vi "Config Trig Template.vi"(4 "Card Position":enum16{"Master", "Slave"}(ring), 6 "Trigger Type":enum16{"Immediate", "Analog Edge"}(ring), 8 "error in (no error)":errorcluster, 11 "4300 in":refnum<class "4300.lvclass">) -> (0 "error out":errorcluster, 3 "4300 out":refnum<class "4300.lvclass">)   [LabVIEW 2016]
uses:
  <resource>/objmgr/daqmx.rc
  Desktop/Built/AnalogInput.lvlibp/AnalogInput.lvclass
  <vilib>/DAQmx/configure/trigger.llb/DAQmx Reference Trigger (Digital Edge).vi
  <vilib>/DAQmx/configure/events/hardwareSignals.llb/DAQmx Export Signal (Most Signals).vi
  <vilib>/DAQmx/configure/trigger.llb/DAQmx Reference Trigger (None).vi
  <vilib>/DAQmx/configure/trigger.llb/DAQmx Reference Trigger (Analog Edge).vi
  4300.lvclass
  C:/Users/rdexter/Desktop/Built/AnalogInput.lvlibp/AnalogInput.lvclass
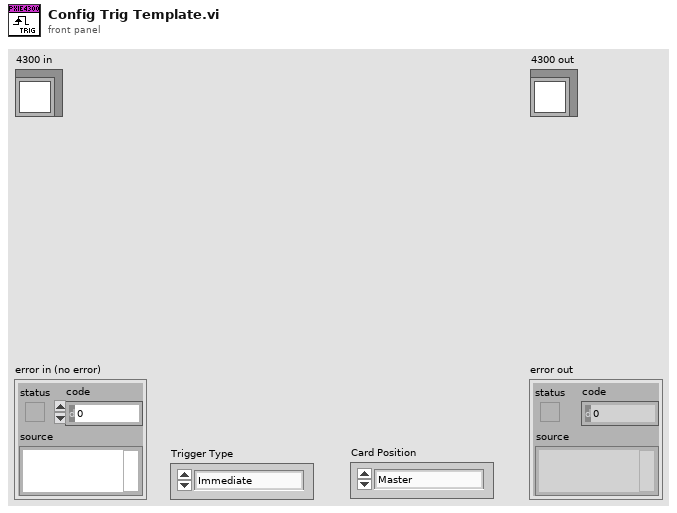
[diagram p1: front panel]
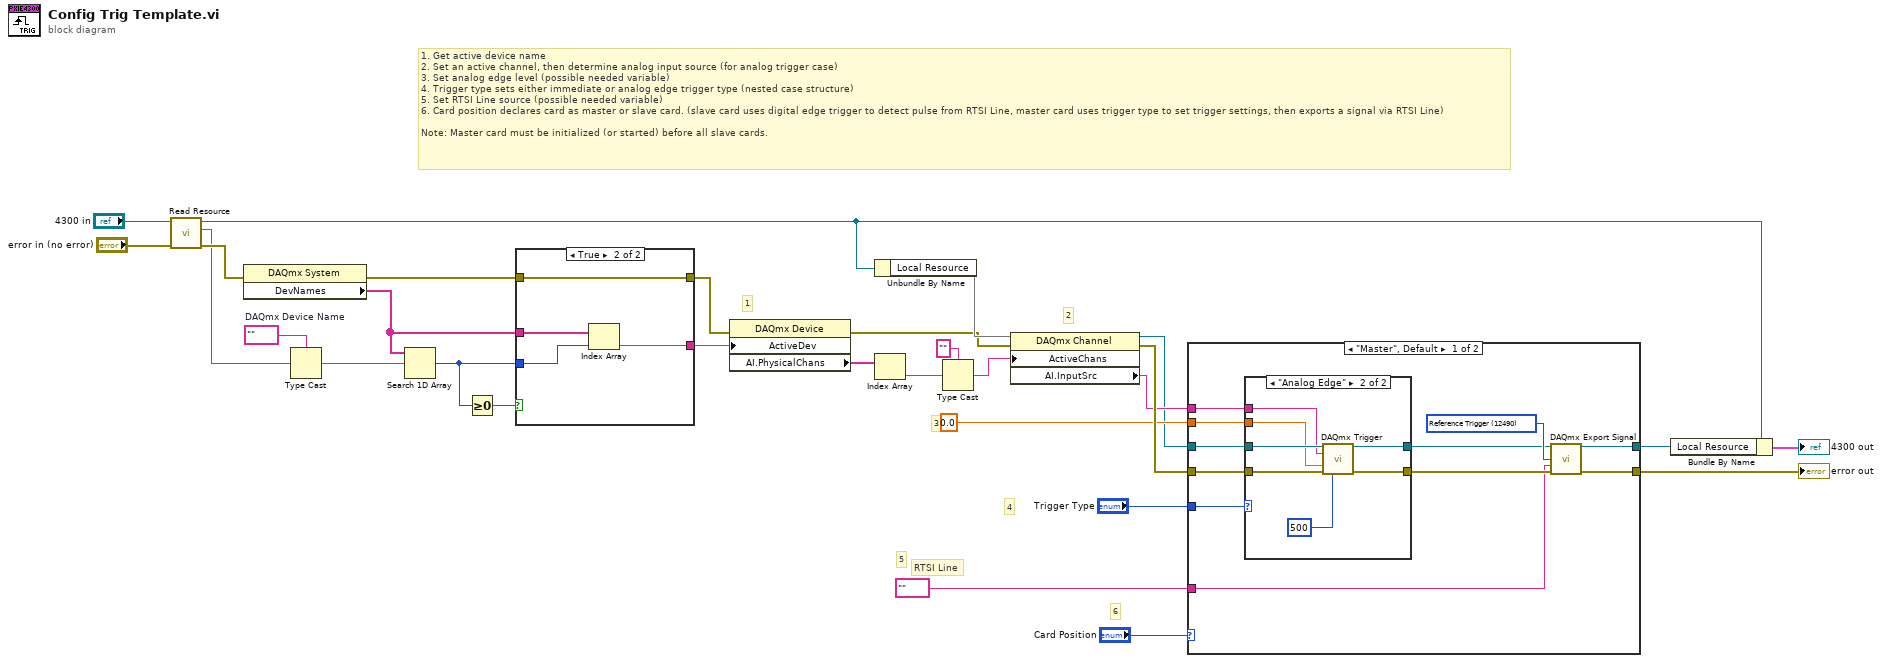
[diagram p0: block diagram]
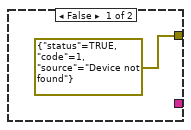
[diagram p2: hidden frame]
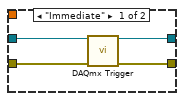
[diagram p3: hidden frame]
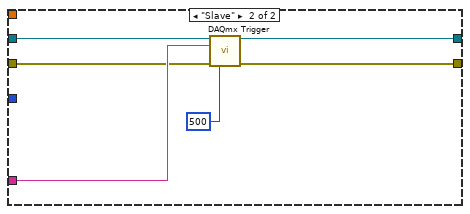
[diagram p4: hidden frame]
diagram:
  w16 = tag ""  # DAQmx Device Name
  # "6"
  # "5"
  # "4"
  # "3"
  # "1. Get active device name\n2. Set an active channel, then determine analog input source (for analog trigger case)\n3. Set analog edge level (possible needed variable)\n4. Trigger type sets either immediate or analog edge trigger type (nested case structure)\n5. Set RTSI Line source (possible needed variable)\n6. Card position declares card as master or slave card. (slave card uses digital edge trigger to detect pulse from RTSI Line, master card uses trigger type to set trigger settings, then exports a signal via RTSI Line)\n\nNote: Master card must be initialized (or started) before all slave cards."
  # "2"
  # "1"
  # "RTSI Line"
  n1 = call "Read Resource.vi"("error in (no error)"="error in (no error)", "AnalogInput in"="4300 in") -> ("error out"=w29:errorcluster, "Resource"=w11:string, "AnalogInput out"=w9:refnum<class "4300.lvclass">)  [unwired: 7 in]
  n2 = property class="DAQmx System"(error in=w29) -> (error out=w12:errorcluster, "DevNames"=w17:tag[])  [unwired: 1 in, 1 out]
  n3 = Type Cast(type=w16, x=w11) -> (*(type *) &x=w15:tag)
  n4 = Search 1D Array(1D array=w17, element=w15) -> (index of element=w13:i32)  [unwired: 1 in]
  n5 = Greater Or Equal To 0?(x=w13) -> (x >= 0?=w14:bool)
  n6 = case shown="True" w14 {
    tunnel: w17 -> [_ w34]
    tunnel: w13 -> [_ w33]
    tunnel: [_ w32] -> w8
    tunnel: w12 -> [_ w31]
    tunnel: [errorcluster {"status"=TRUE, "code"=1, "source"="Device not found"} ("error out") w31] -> w6
    frame False {
    }
    frame True {
      n7 = Index Array(array=w34, index=w33) -> (element=w32:tag)
    }
  }
  n8 = property class="DAQmx Device"(error in=w6, "ActiveDev"=w8) -> (error out=w5:errorcluster, "AI.PhysicalChans"=w18:tag[])  [unwired: 1 in, 1 out]
  n9 = Unbundle By Name(w9) -> ("Local Resource"=w23)
  n10 = Index Array(array=w18) -> (element=w25:tag)  [unwired: 1 in]
  n11 = Type Cast(type="", x=w25) -> (*(type *) &x=w19:string)
  n12 = property class="DAQmx Channel"(reference=w23, error in=w5, "ActiveChans"=w19) -> (reference out=w4:refnum<k21>, error out=w28:errorcluster, "AI.InputSrc"=w20:string)
  n13 = case shown="\"Master\", Default" "Card Position" {
    tunnel: w4 -> [w44 w62]
    tunnel: tag "" ("source") -> [w35 w61]
    tunnel: [w36 w60] -> w27
    tunnel: [w37 w59] -> w22
    tunnel: w28 -> [w43 w58]
    tunnel: 0.0 -> [w41 _]
    tunnel: w20 -> [w42 _]
    tunnel: "Trigger Type" -> [w45 _]
    frame "Master", Default {
      w40 = 12490 items=["AI Convert Clock"=12484, "10MHz Reference Clock"=12536, "20MHz Timebase Clock"=12486, "Sample Clock"=12487, "Advance Trigger"=12488, "Reference Trigger"=12490, "Start Trigger"=12491, "Advance Complete Event"=12492, "AI Hold Complete Event"=12493, "Counter Output Event"=12494, "Change Detection Event"=12511, "Watchdog Timer Expired Event"=12512] ("signal")
      n14 = case shown="\"Analog Edge\"" w45 {
        tunnel: w44 -> [w49 w55]
        tunnel: w43 -> [w48 w54]
        tunnel: w42 -> [_ w52]
        tunnel: w41 -> [_ w53]
        tunnel: [w47 w51] -> w38
        tunnel: [w46 w50] -> w39
        frame "Immediate" {
          n15 = call-poly <vilib>:"DAQmx Trigger.vi"("task/channels in"=w49, "error in"=w48) -> ("task out"=w47:refnum<k21>, "error out"=w46:errorcluster)  [unwired: 12 in]
        }
        frame "Analog Edge" {
          n16 = call-poly <vilib>:"DAQmx Trigger.vi"("task/channels in"=w55, "source"=w52, "level"=w53, "error in"=w54, "pretrigger samples per channel"=u32 500) -> ("task out"=w51:refnum<k21>, "error out"=w50:errorcluster)  [unwired: 9 in]
        }
      }
      n17 = call-poly <vilib>:"DAQmx Export Signal.vi"("task/channels in"=w38, "signal"=w40, "output terminal"=w35, "error in"=w39) -> ("task out"=w37:refnum<k21>, "error out"=w36:errorcluster)  [unwired: 10 in]
    }
    frame "Slave" {
      n18 = call-poly <vilib>:"DAQmx Trigger.vi"("task/channels in"=w62, "source"=w61, "error in"=w58, "pretrigger samples per channel"=u32 500) -> ("task out"=w59:refnum<k21>, "error out"=w60:errorcluster)  [unwired: 10 in]
    }
  }
  "error out" <- w27
  n19 = Bundle By Name(cluster=w9, "Local Resource"=w22) -> (→"4300 out":cluster{})
